vi "4_Rx_DSB_AM.vi"() -> ()   [LabVIEW 2022 SP3]
uses:
  <instrlib>/niUSRP/niUSRP Fetch Rx Data (CDB WDT).vi
panel:
  in  "device names":refnum<k15>
  in  "Amplitude":dbl=1.0
  out "Demodulated\nDSB-AM":dynamicdata(graph) caption="Filtered Signal"
  out "error out":errorcluster
  in  "stop":bool
  out "Waveform Graph":dbl[](graph)
  in  "active antenna":string
  in  "gain":dbl format="%#_6f"
  in  "carrier frequency":dbl=100000.0 format="%#_6p"
  in  "IQ rate":dbl=100000.0 format="%#_6p"
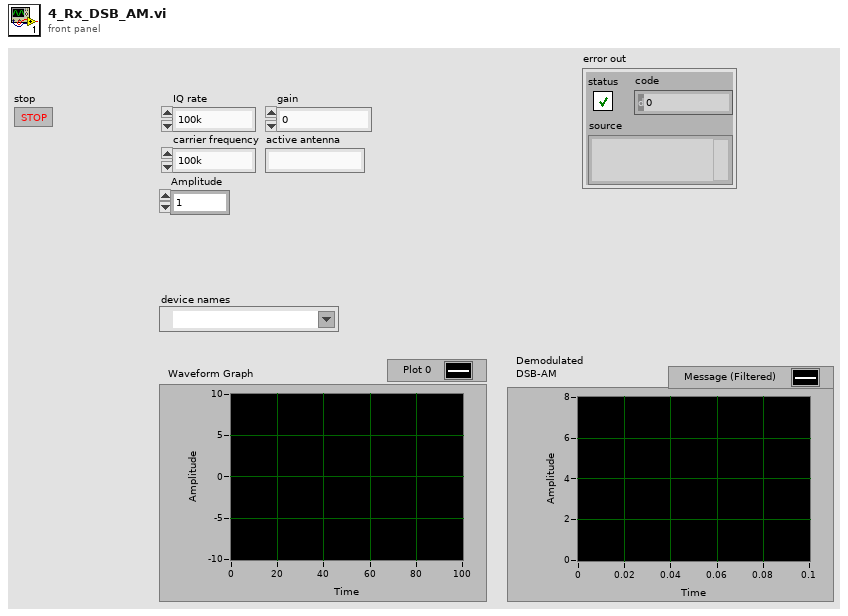
[diagram p1: front panel]
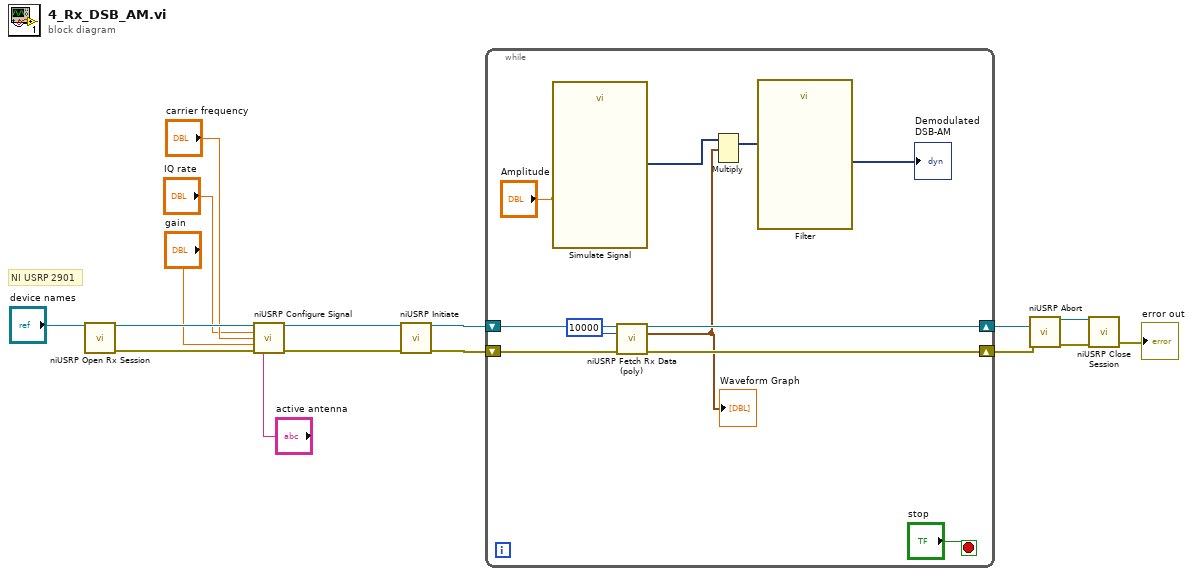
[diagram p0: block diagram]
diagram:
  # "NI USRP 2901"
  n1 = call <instrlib>:"niUSRP Open Rx Session.vi"("device names"="device names") -> ("session handle out"=w9:refnum<k15>, "error out"=w8:errorcluster)  [unwired: 13 in]
  n2 = call <instrlib>:"niUSRP Configure Signal.vi"("session handle"=w9, "IQ rate"="IQ rate", "carrier frequency"="carrier frequency", "gain"="gain", "error in (no error)"=w8, "active antenna"="active antenna") -> ("session handle out"=w7:refnum<k15>, "error out"=w14:errorcluster)  [unwired: 5 in, 3 out]
  n3 = call <instrlib>:"niUSRP Initiate.vi"("session handle"=w7, "error in (no error)"=w14) -> ("session handle out"=w13:refnum<k15>, "error out"=w12:errorcluster)  [unwired: 12 in]
  n4 = while {
    shift-right: [w25] -> w11
    shift-left: w13 -> [w27]
    shift-right: [w22] -> w10
    shift-left: w12 -> [w26]
    stop <- "stop" stop-if-true
    n5 = call "Simulate Signal"("Amplitude"="Amplitude") -> ("Carrier"=w18:dynamicdata)  [unwired: 13 in, 1 out]
    n6 = call-poly <instrlib>:"niUSRP Fetch Rx Data (poly).vi"("session handle"=w27, "number of samples"=i64 10000, "error in (no error)"=w26) -> ("session handle out"=w25:refnum<k15>, "data"=w20:waveform(cdb), "error out"=w22:errorcluster)  [unwired: 9 in, 1 out]
    "Waveform Graph" <- w20
    n7 = Multiply(1:w20, 2:w18) -> (0:w17:dynamicdata)  [unwired: 1 in, 1 out]
    n8 = call "Filter"("Signal"=w17) -> ("Filtered Signal"=→"Demodulated\nDSB-AM":dynamicdata)  [unwired: 9 in, 1 out]
  }
  n9 = call <instrlib>:"niUSRP Abort.vi"("session handle"=w11, "error in (no error)"=w10) -> ("session handle out"=w16:refnum<k15>, "error out"=w15:errorcluster)  [unwired: 12 in]
  n10 = call <instrlib>:"niUSRP Close Session.vi"("session handle"=w16, "error in (no error)"=w15) -> ("error out"=→"error out":errorcluster)  [unwired: 13 in]
